vi "Material-ConfigDialog-DiscoverPages.vi"(7 "Custom Config Pages Directory":path, 11 "error in":errorcluster) -> (4 "Configuration Dialog Page Filepaths":path[](array[path]), 6 "Display Names":string[](array[string]), 8 "Descriptions":string[](array[string]), 10 "Tree Tags":string[](array[string]), 15 "error out":errorcluster)   [LabVIEW 2013, in "Material-ConfigDialog.lvclass"]
uses:
  Material-ConfigDialog.lvclass
  Deploy Application/Material-Application-Constants.vi
panel:
  # "Inputs"
  # "Outputs"
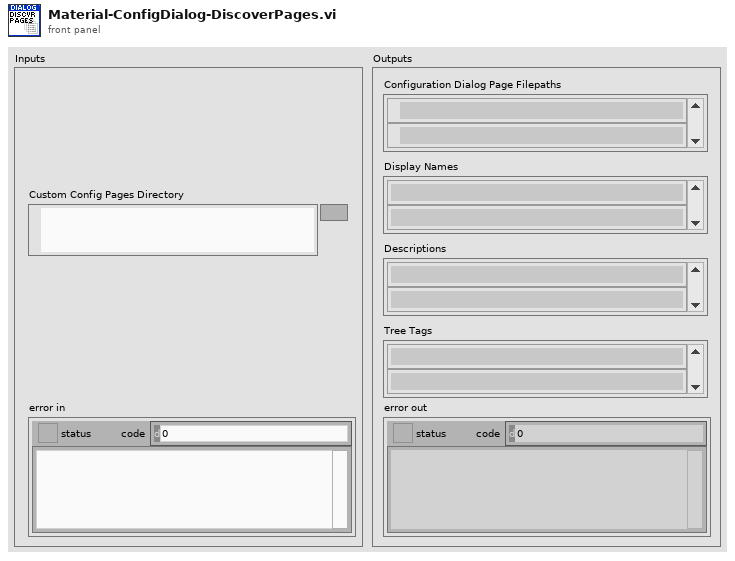
[diagram p1: front panel]
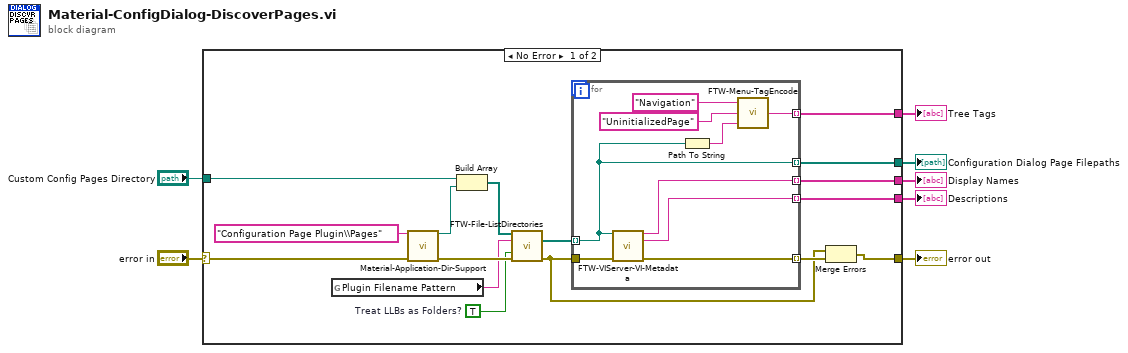
[diagram p0: block diagram]
diagram:
  n1 = case shown="No Error" "error in" {
    selector: "error in" -> [w21 w33]
    tunnel: [w16 w33] -> w7
    tunnel: [w18 _] -> w5
    tunnel: "Custom Config Pages Directory" -> [w22 _]
    tunnel: [w15 _] -> w3
    tunnel: [w14 _] -> w2
    tunnel: [w13 _] -> w1
    frame No Error {
      w9 = TRUE  # Treat LLBs as Folders?
      n2 = global read "Material-Application-Constants.vi" "Plugin Filename Pattern"() -> (w8:string)
      n3 = call "Material-Application-Dir-Support.vi"("Support Resource Relative Filepath"="Configuration Page Plugin\\Pages" ("Support VI Relative Filepath"), "error in"=w21) -> ("Support Filepath"=w10:path, "error out"=w20:errorcluster)  [unwired: 12 in]
      n4 = Build Array(w22, w10) -> (w23:path[])
      n5 = call "FTW-File-ListDirectories.vi"("Directories"=w23, "Matching Filename Pattern"=w8, "Treat LLBs as Folders?"=w9, "error in"=w20) -> ("Matching Filepaths"=w11:path[], "error out"=w17:errorcluster)  [unwired: 9 in, 1 out]
      n6 = for {
        tunnel: w11 -> [w25] mode=indexing
        tunnel: [w32] -> w15 mode=indexing
        tunnel: w17 -> [w31]
        tunnel: [w30] -> w19 mode=indexing
        tunnel: [w29] -> w14 mode=indexing
        tunnel: [w24] -> w13 mode=indexing
        tunnel: [w25] -> w18 mode=indexing
        n7 = call "FTW-VIServer-VI-Metadata.vi"("VI Filepath"=w25, "error in"=w31) -> ("Front Panel Title"=w32:string, "VI Description"=w29:string, "error out"=w30:errorcluster)  [unwired: 11 in]
        n8 = Path To String(path=w25) -> (string=w27:string)
        n9 = call "FTW-Menu-TagEncode.vi"("Payload"=w27, "Command"="UninitializedPage", "Class"="Navigation") -> ("Tag"=w24:string)  [unwired: 1 in]
      }
      n10 = Merge Errors(w17, w19) -> (w16:errorcluster)
    }
    frame Error {
    }
  }
  "error out" <- w7
  "Configuration Dialog Page Filepaths" <- w5
  "Tree Tags" <- w1
  "Display Names" <- w3
  "Descriptions" <- w2
